vi "date_hour.vi"(3 "Array":timestamp[](array[timestamp])) -> (0 "date/hour":timestamp[](array[timestamp]), 1 "appended array":string[][](array[string]))   [LabVIEW 2017]
panel:
  in  "Array 2":string[](array[string])=["fecha", "hora"]
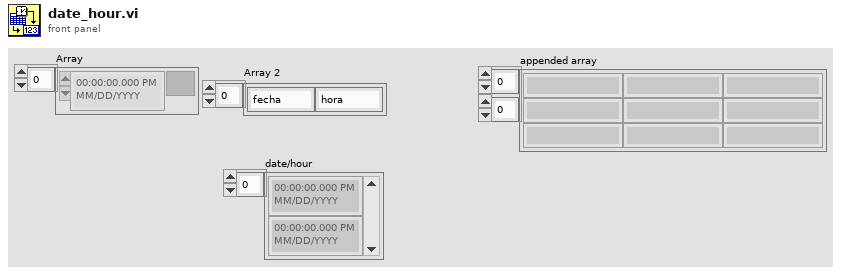
[diagram p1: front panel]
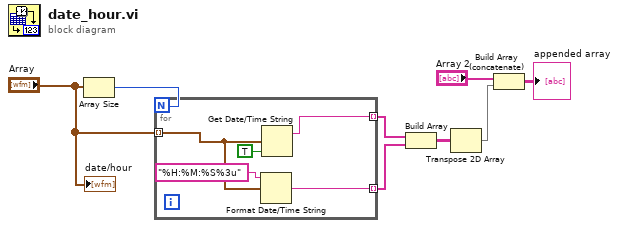
[diagram p0: block diagram]
diagram:
  n1 = Array Size(array="Array") -> (size(s)=w5:i32)
  n2 = for {
    N: w5 -> [_]
    tunnel: "Array" -> [w11] mode=indexing
    tunnel: [w13] -> w7 mode=indexing
    tunnel: [w9] -> w1 mode=indexing
    n3 = Format Date/Time String(time format string (%c)="%H:%M:%S%3u", seconds (now)=w11) -> (date/time string=w9:string)  [unwired: 1 in]
    n4 = Get Date/Time String(seconds (now)=w11, want seconds? (F)=TRUE) -> (date string=w13:string)  [unwired: 1 in, 1 out]
  }
  n5 = Build Array(w7, w1) -> (w8:string[][])
  n6 = Transpose 2D Array(2D array=w8) -> (transposed array=w3:string[][])
  n7 = Build Array (concatenate)("Array 2", w3) -> (→"appended array":string[][])
  "date/hour" <- "Array"
